vi "亚为噪音 例子.vi"() -> ()   [LabVIEW 2011]
panel:
  out "Max":dbl format="%_4f"
  out "Min":dbl format="%_4f"
  out "?":cluster{dbl, dbl, dbl}(knob)={0.0, 30.0, 30.0} scale=30.0..130.0
  out "波形图表 2":dbl(graph)
  out "s? t:f":dbl
  out "子数组 2":dbl[](array[numeric])
  in  "采样率":u16(ring)=2 items=["200Hz", "500Hz", "1KHz", "2KHz", "5KHz", "10KHz", "20KHz", "50KHz", "100KHz", "200KHz"]
  in  "id":u16
  out "波形图表":dbl[][](graph)
  out "错误输出":errorcluster
  out "设备":string[](array[string])
  out "已强制转换(x)":dbl
  in  "Duration (ms)":u16=100 min=200 max=10000 step=100
  in  "Device":u32 caption="设备"
  out "数组 2":dbl[](array[numeric])
  in  "数值 3":dbl
  in  "数值 2":dbl
  in  "退出":bool
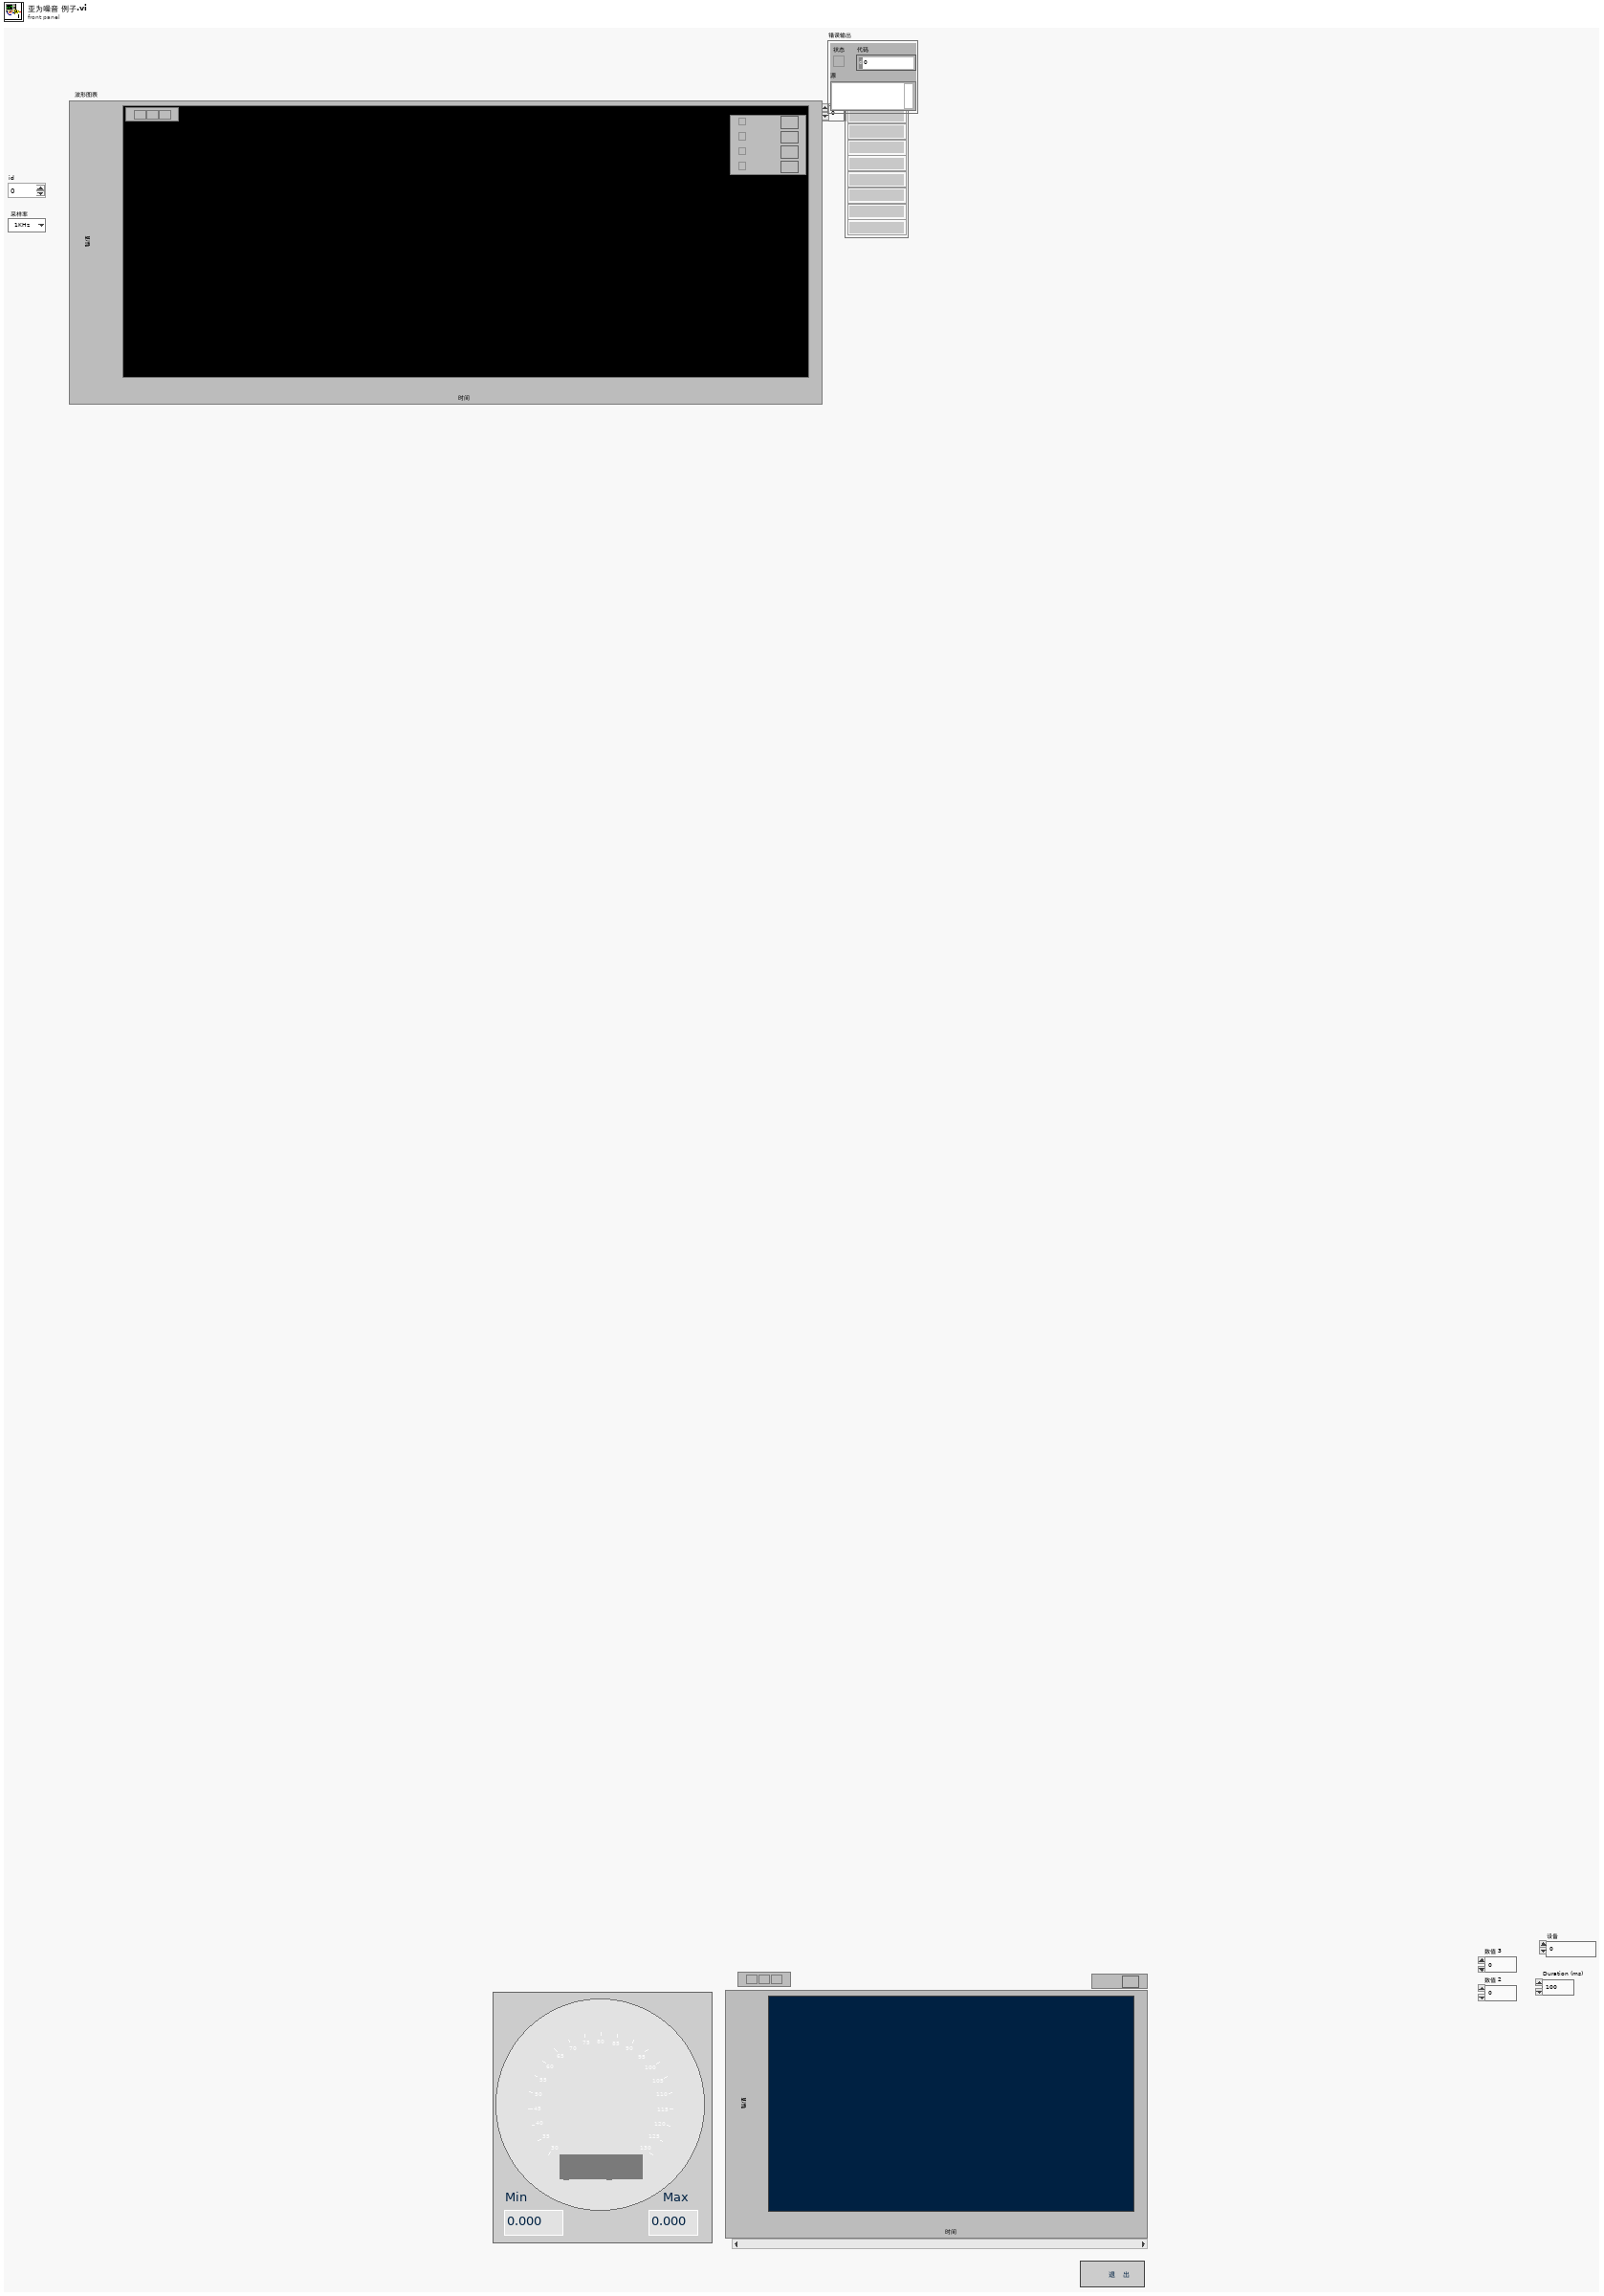
[diagram p1: front panel]
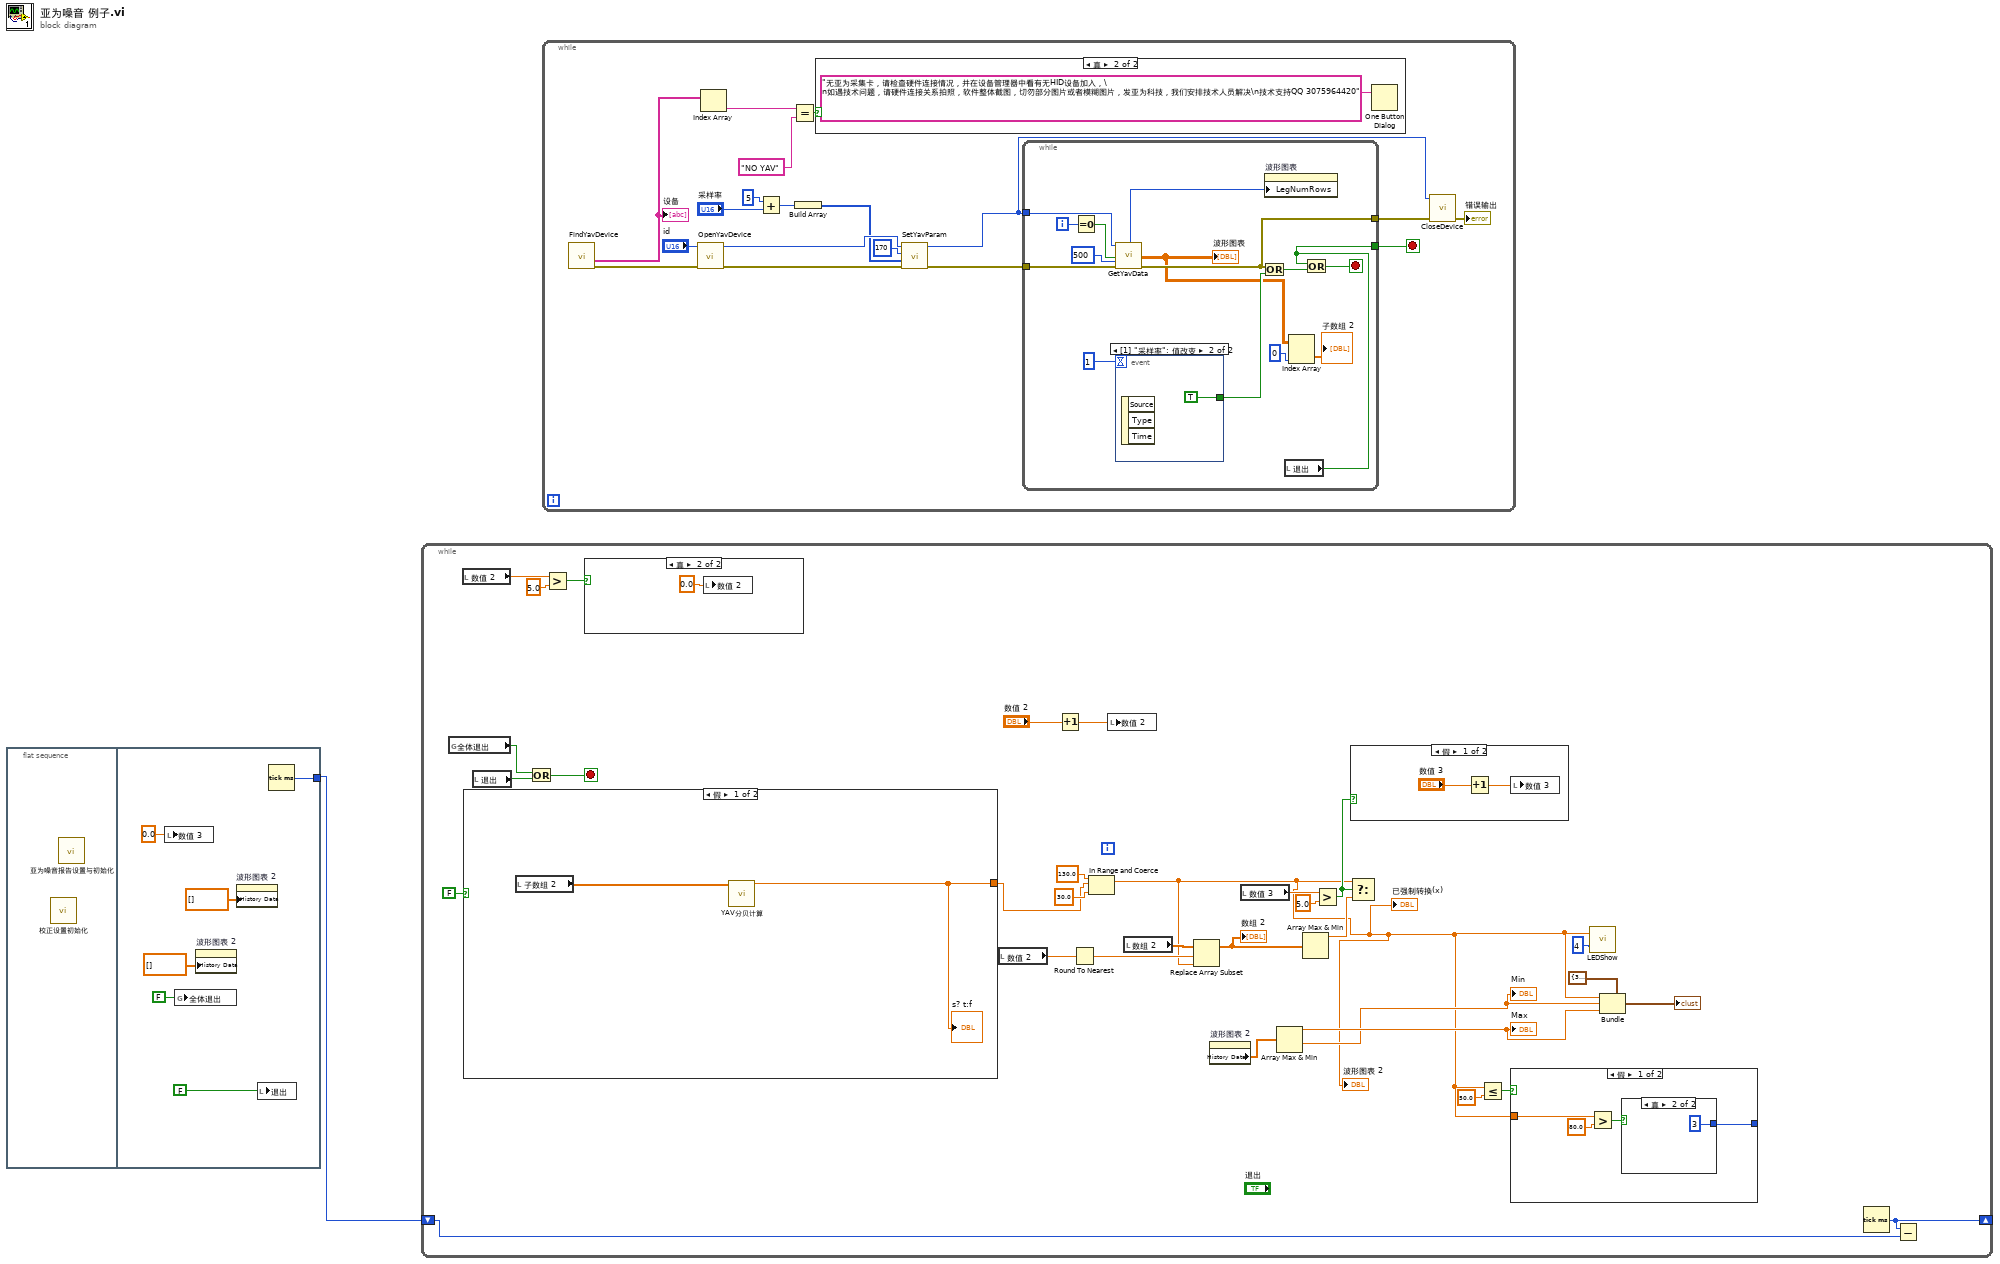
[diagram p0: block diagram]
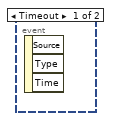
[diagram p3: hidden frame]
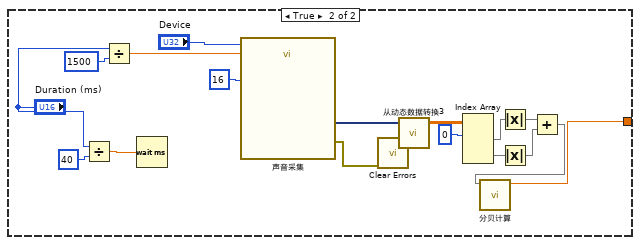
[diagram p4: hidden frame]
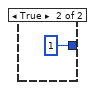
[diagram p6: hidden frame]
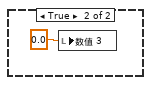
[diagram p8: hidden frame]
diagram:
  n1 = flat-sequence {
    tunnel: [w7] -> w1
    frame #0 {
      n2 = call "校正设置初始化.vi"() -> ()  [unwired: 11 in, 1 out]
      n3 = call "亚为噪音报告设置与初始化.vi"() -> ()  [unwired: 11 in, 1 out]
    }
    frame #1 {
      n4 = local write "数值 3"(0.0 ("数值")) -> ()
      n5 = global write "全局变量.vi" "全体退出"(FALSE ("全体退出")) -> ()
      n6 = property on="波形图表 2" class="WFChart (严格)"("History Data"=dbl[] [] ("历史数据")) -> ()  [unwired: 2 in, 2 out]
      n7 = property on="波形图表 2" class="WFChart (严格)"("History Data"=dbl[] [] ("历史数据")) -> ()  [unwired: 2 in, 2 out]
      n8 = local write "退出"(FALSE ("退出")) -> ()
      n9 = Tick Count (ms)() -> (millisecond timer value=w7:u32)
    }
  }
  n10 = while {
    shift-right: [w23] -> _
    shift-left: w1 -> [w22]
    stop <- w20 stop-if-true
    n11 = global read "全局变量.vi" "全体退出"() -> (w19:bool)
    n12 = local read "数值 2"() -> (w30:dbl)
    n13 = case shown="假" FALSE {
      tunnel: [w39 w41] -> w15
      frame False {
        n14 = local read "子数组 2"() -> (w40:dbl[])
        n15 = call "YAV分贝计算.vi"("子数组输入"=w40) -> ("f"=w39:dbl)  [unwired: 10 in]
        "s? t:f" <- w39
      }
      frame True {
        n16 = Divide(x="Duration (ms)", y=u16 40) -> (x/y=w43:dbl)
        n17 = Divide(x="Duration (ms)", y=u16 1500) -> (x/y=w48:dbl)
        n18 = Wait (ms)(milliseconds to wait=w43) -> ()  [unwired: 1 out]
        n19 = call "声音采集"("Device"="Device", "Duration (s)"=w48, "Resolution (bits)"=16) -> ("Data"=w51:dynamicdata, "error out"=w46:errorcluster)  [unwired: 15 in]
        n20 = call <vilib>:"Clear Errors.vi"("error in (no error)"=w46) -> ()  [unwired: 5 in, 2 out]
        n21 = call "从动态数据转换3"("Dynamic Data Type"=w51) -> ("Array"=w52:dbl[][])  [unwired: 3 in]
        n22 = Index Array(array=w52, index (row) #1=0 ("索引 (行)")) -> (element #1=w53:dbl[], element #2=w55:dbl[])  [unwired: 3 in]
        n23 = Absolute Value(x=w53) -> (abs(x)=w57:dbl[])
        n24 = Absolute Value(x=w55) -> (abs(x)=w56:dbl[])
        n25 = Add(x=w57, y=w56) -> (x+y=w42:dbl[])
        n26 = call "分贝计算.vi"("数组"=w42) -> ("数值"=w41:dbl)  [unwired: 10 in]
      }
    }
    n27 = local read "退出"() -> (w26:bool)
    n28 = Or(x=w19, y=w26) -> (x .or. y?=w20:bool)
    n29 = Greater?(x=w30, y=5.0) -> (0:w27:bool)
    n30 = case shown="真" w27 {
      frame False {
      }
      frame True {
        n31 = local write "数值 2"(0.0 ("数值 2")) -> ()
      }
    }
    n32 = local read "数值 2"() -> (w28:dbl)
    n33 = Increment(x="数值 2") -> (x+1=w31:dbl)
    n34 = Round To Nearest(number=w28) -> (nearest integer value=w37:dbl)
    n35 = In Range and Coerce(upper limit=130.0 ("上限"), x=w15, lower limit=30.0 ("下限")) -> (coerced(x)=w11:dbl)  [unwired: 1 out]
    "已强制转换(x)" <- w11
    "波形图表 2" <- w11
    n36 = local write "数值 2"(w31) -> ()
    n37 = local read "数组 2"() -> (w38:dbl[])
    n38 = Replace Array Subset(array=w38, new element=w11, index=w37) -> (w13:dbl[])
    "数组 2" <- w13
    n39 = property on="波形图表 2" class="WFChart (严格)"() -> ("History Data"=w14:dbl[])  [unwired: 2 in, 2 out]
    n40 = local read "数值 3"() -> (w34:dbl)
    n41 = Array Max & Min(array=w14) -> (max value=w21:dbl, min value=w12:dbl)  [unwired: 2 out]
    "Max" <- w21
    "Min" <- w12
    n42 = Array Max & Min(array=w13) -> (max value=w33:dbl)  [unwired: 3 out]
    n43 = Greater?(x=w34, y=5.0) -> (0:w35:bool)
    n44 = case shown="假" w35 {
      frame False {
        n45 = Increment(x="数值 3") -> (x+1=w65:dbl)
        n46 = local write "数值 3"(w65) -> ()
      }
      frame True {
        n47 = local write "数值 3"(0.0) -> ()
      }
    }
    n48 = Select(t=w11, s=w35, f=w33) -> ()  [unwired: 1 out]
    n49 = Less Or Equal?(x=w11, y=50.0) -> (x <= y?=w24:bool)
    n50 = case shown="假" w24 {
      tunnel: [w58 1] -> _
      tunnel: w11 -> [w59 _]
      frame False {
        n51 = Greater?(x=w59, y=80.0) -> (0:w61:bool)
        n52 = case shown="真" w61 {
          tunnel: [_ 3] -> w58
          frame False {
          }
          frame True {
          }
        }
      }
      frame True {
      }
    }
    n53 = call "LEDShow.vi"("DigntNumber"=u32 4, "InputNumber"=w11) -> ()  [unwired: 1 out]
    n54 = Bundle(cluster=cluster{dbl, dbl, dbl} {30.0, 30.0, 30.0} ("量表 2"), w11, w12, w21) -> (→"?":cluster{dbl, dbl, dbl})
    n55 = Tick Count (ms)() -> (millisecond timer value=w23:u32)
    n56 = Subtract(x=w23, y=w22) -> ()  [unwired: 1 out]
  }
  n57 = while {
    stop <- w75 stop-if-true
    n58 = call "FindYavDevice.vi"() -> ("错误输出"=w85:errorcluster, "设备"=w71:string[])  [unwired: 9 in, 1 out]
    "设备" <- w71
    n59 = call "OpenYavDevice.vi"("错误输入（无错误）"=w85, "ID"="id") -> ("错误输出"=w81:errorcluster, "ID"=w82:u32)  [unwired: 8 in]
    n60 = Index Array(array=w71) -> (element=w70:string)  [unwired: 1 in]
    n61 = Add(x=u16 5, y="采样率") -> (x+y=w78:u16)
    n62 = Equal?(x=w70, y="NO YAV") -> (x = y?=w68:bool)
    n63 = Build Array(w78) -> (w73:u16[])
    n64 = case shown="真" w68 {
      frame False {
      }
      frame True {
        n65 = One Button Dialog(message="无亚为采集卡，请检查硬件连接情况，并在设备管理器中看有无HID设备加入，\n如遇技术问题，请硬件连接关系拍照，软件整体截图，切勿部分图片或者模糊图片，发亚为科技，我们安排技术人员解决\n技术支持QQ 3075964420" ("消息")) -> ()  [unwired: 1 in, 1 out]
      }
    }
    n66 = call "SetYavParam.vi"("错误输入（无错误）"=w81, "WriteParam"=w73, "CMD"=u8 170, "ID"=w82) -> ("错误输出"=w84:errorcluster, "ID"=w76:u32)  [unwired: 6 in]
    n67 = while {
      tunnel: w84 -> [w101]
      tunnel: w76 -> [w100]
      tunnel: [w95] -> w77
      tunnel: [w87] -> w75
      i -> [w93]
      stop <- w94 stop-if-true
      n68 = Equal To 0?(x=w93) -> (x = 0?=w92:bool)
      n69 = call "GetYavData.vi"("ID"=w100, "初始化"=w92, "采样长度"=500, "错误输入（无错误）"=w101) -> ("通道数"=w91:i32, "数组 列通道号"=w90:dbl[][], "error out"=w95:errorcluster)  [unwired: 4 in, 9 out]
      "波形图表" <- w90
      n70 = event shown="[1] \"采样率\": 值改变" {
        selector: _ -> [_ _]
        dyn-events: _ -> [_ _]
        timeout: 1 -> [_ _]
        tunnel: [_ TRUE] -> w97
        event Timeout {
          n71 = event-data() -> ()  [unwired: 1 in, 3 out]
        }
        event "采样率": Value Change {
          n72 = event-data() -> ()  [unwired: 1 in, 3 out]
        }
      }
      n73 = Or(x=w95, y=w97) -> (x .or. y?=w98:bool)
      n74 = property on="波形图表" class="WFChart (严格)"("LegNumRows"=w91) -> ()  [unwired: 2 in, 2 out]
      n75 = local read "退出"() -> (w87:bool)
      n76 = Index Array(array=w90, index (col)=0 ("索引 (行)")) -> (element=→"子数组 2":dbl[])  [unwired: 1 in]
      n77 = Or(x=w87, y=w98) -> (x .or. y?=w94:bool)
    }
    n78 = call "CloseDevice.vi"("error in (no error)"=w77, "id"=w76) -> ("错误输出"=→"错误输出":errorcluster)  [unwired: 9 in]
  }
